vi "ChngGrphWindow.vi"(8 "error in (no error)":errorcluster caption="entrée d'erreur (pas d'erreur)", 9 "NewGraphInd":i32, 10 "CurvesIndx":i32[](array[numeric]), 11 "Interface en entrée":refnum<class "Interface.lvclass"> caption="DNL_LabVIEW Object in") -> (0 "error out":errorcluster caption="sortie d'erreur", 3 "Interface en sortie":refnum<class "Interface.lvclass"> caption="DNL_LabVIEW Object out")   [LabVIEW 2010, in "Interface.lvclass"]
uses:
  Interface.lvclass
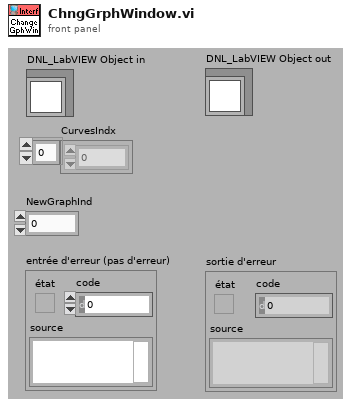
[diagram p1: front panel]
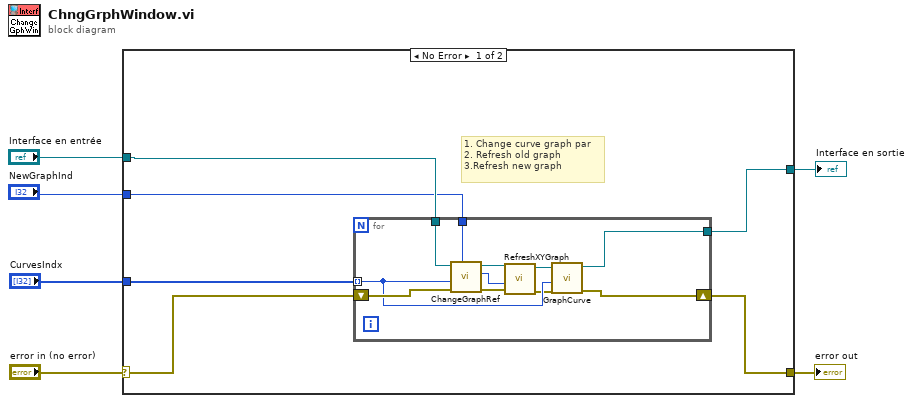
[diagram p0: block diagram]
diagram:
  n1 = case shown="No Error" "error in (no error)" {
    selector: "error in (no error)" -> [w7 w25]
    tunnel: [w11 w25] -> w5
    tunnel: [w10 w24] -> w3
    tunnel: "Interface en entrée" -> [w9 w24]
    tunnel: "CurvesIndx" -> [w12 _]
    tunnel: "NewGraphInd" -> [w8 _]
    frame No Error {
      # "1. Change curve graph par\n2. Refresh old graph\n3.Refresh new graph"
      n2 = for {
        tunnel: w12 -> [w18] mode=indexing
        tunnel: w9 -> [w22]
        shift-right: [w21] -> w11
        shift-left: w7 -> [w23]
        tunnel: [w20] -> w10
        tunnel: w8 -> [w19]
        n3 = call "ChangeGraphRef.vi"("NewGraphIndex"=w19, "error in (no error)"=w23, "CurveIndex"=w18, "Interface en entrée"=w22) -> ("error out"=w14:errorcluster, "OldGraphIndex"=w13:i32, "Interface en sortie"=w15:refnum<class "Interface.lvclass">)  [unwired: 5 in]
        n4 = call "RefreshXYGraph.vi"("error in (no error)"=w14, "Graph Index"=w13, "Interface en entrée"=w15) -> ("error out"=w17:errorcluster, "Interface en sortie"=w16:refnum<class "Interface.lvclass">)  [unwired: 5 in, 2 out]
        n5 = call "GraphCurve.vi"("error in (no error)"=w17, "CurvIndex"=w18, "Interface en entrée"=w16) -> ("error out"=w21:errorcluster, "Interface en sortie"=w20:refnum<class "Interface.lvclass">)  [unwired: 7 in]
      }
    }
    frame Error {
    }
  }
  "error out" <- w5
  "Interface en sortie" <- w3
